vi "Initialize.vi"(0 "BroadcastRegistry in":refnum<class "BroadcastRegistry.lvclass">) -> (4 "BroadcastRegistry out":refnum<class "BroadcastRegistry.lvclass">)   [LabVIEW 2020, in "Communicable State Machine.lvlib" / "BroadcastRegistry.lvclass"]
uses:
  BroadcastRegistry.lvclass
  BroadcastRegistry.lvclass/BroadcastRegistry.ctl
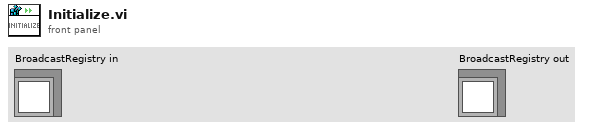
[diagram p1: front panel]
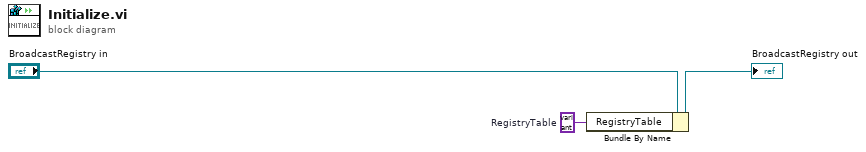
[diagram p0: block diagram]
diagram:
  w1 = variant  # RegistryTable
  n1 = Bundle By Name(cluster="BroadcastRegistry in", "RegistryTable"=w1) -> (→"BroadcastRegistry out":refnum<class "BroadcastRegistry.lvclass">)
